vi "ma_check Time History Signal Continuity.vi"(4 "dt":dbl format="%0.2f", 6 "t0":timestamp format="%<%.4X>T", 7 "Ignore input start time":bool, 8 "error in (no error)":errorcluster, 9 "# samples":i32, 11 "state info":T1 {"buffer" format="%0.2f"; "timestamp" format="%<%.4X>T"; "dt history" format="%0.2f"; "t0 history" format="%<%I:%M:%S%4u %p>T"; "exp TC (samples)" format="%0.2f"; "RMS history" format="%0.2f"; "DC history" format="%0.2f"}) -> (0 "error out":errorcluster, 1 "dt changed":bool, 2 "t0 changed":bool, 3 "state info":T1 {"buffer" format="%0.2f"; "timestamp" format="%<%.4X>T"; "dt history" format="%0.2f"; "t0 history" format="%<%I:%M:%S%4u %p>T"; "exp TC (samples)" format="%0.2f"; "RMS history" format="%0.2f"; "DC history" format="%0.2f"}, 5 "epsilon used":dbl format="%0.2f")   [LabVIEW 2022 SP3, in "NI_MAPro.lvlib"]
uses:
  NI_MAPro.lvlib
  NI_MABase.lvlib
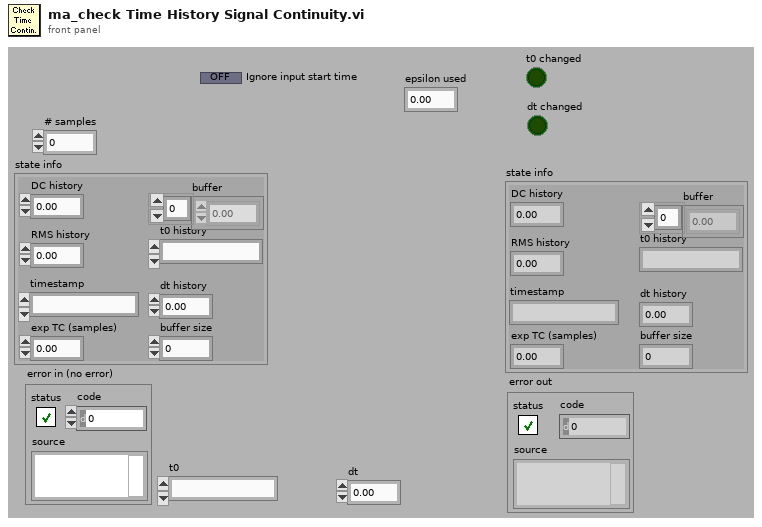
[diagram p1: front panel]
types:
  T1 = cluster{"DC history":dbl, "RMS history":dbl, "exp TC (samples)":dbl, "buffer size":i32, "t0 history":timestamp, "dt history":dbl, "timestamp":timestamp, "buffer":dbl[]}
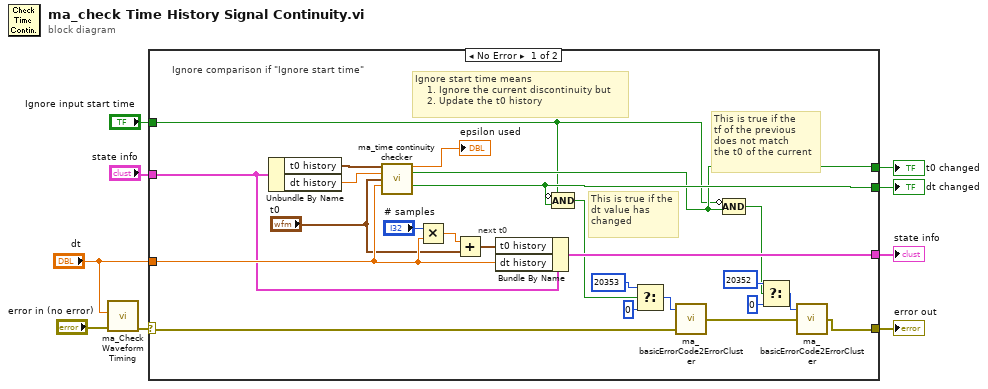
[diagram p0: block diagram]
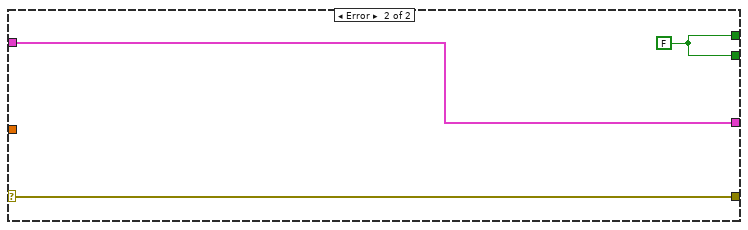
[diagram p2: hidden frame]
diagram:
  n1 = call "ma_Check Waveform Timing.vi"("error in (no error)"="error in (no error)", "dt"="dt") -> ("error out"=w3:errorcluster)  [unwired: 8 in, 1 out]
  n2 = case shown="No Error" w3 {
    selector: w3 -> [w29 w34]
    tunnel: [w33 w34] -> w2
    tunnel: [w13 w36] -> w9
    tunnel: [w14 w36] -> w8
    tunnel: [w32 w35] -> w7
    tunnel: "dt" -> [w31 _]
    tunnel: "state info" -> [w30 w35]
    tunnel: "Ignore input start time" -> [w12 _]
    frame No Error {
      # "Ignore start time means \n    1. Ignore the current discontinuity but\n    2. Update the t0 history"
      # "next t0"
      # "This is true if the\ntf of the previous\ndoes not match \nthe t0 of the current"
      # "This is true if the\ndt value has \nchanged"
      # "Ignore comparison if \"Ignore start time\""
      n3 = Unbundle By Name(w30) -> ("t0 history"=w21:timestamp, "dt history"=w18:dbl)
      n4 = call "ma_time continuity checker.vi"("timestamp previous"=w21, "dt previous"=w18, "timestamp current"="t0", "dt current"=w31) -> ("epsilon used"=→"epsilon used":dbl, "t0 changed"=w13:bool, "dt changed"=w14:bool)  [unwired: 8 in, 1 out]
      n5 = Multiply(x="# samples", y=w31) -> (x*y=w17:dbl)
      n6 = Add(x=w17, y="t0") -> (x+y=w15:timestamp)
      n7 = Bundle By Name(cluster=w30, "t0 history"=w15, "dt history"=w31) -> (w32:T1)
      n8 = Compound Arithmetic op=AND(invert w12, w14) -> (w11:bool)
      n9 = Select(t=20353 ("code"), s=w11, f=0) -> (s? t:f=w24:i32)
      n10 = call "ma_basicErrorCode2ErrorCluster.vi"("error in (no error)"=w29, "Error Code"=w24) -> ("error out"=w23:errorcluster)  [unwired: 1 in]
      n11 = Compound Arithmetic op=AND(invert w12, w13) -> (w10:bool)
      n12 = Select(t=20352 ("code"), s=w10, f=0) -> (s? t:f=w22:i32)
      n13 = call "ma_basicErrorCode2ErrorCluster.vi"("error in (no error)"=w23, "Error Code"=w22) -> ("error out"=w33:errorcluster)  [unwired: 1 in]
    }
    frame Error {
      w36 = FALSE ("t0 changed")
    }
  }
  "error out" <- w2
  "dt changed" <- w8
  "t0 changed" <- w9
  "state info" <- w7
